vi "OpenTextFile.vi"(4 "Sequence Context":T1) -> (0 "error out":errorcluster, 1 "Test Data":T2 {"Numeric Measurement" format="%.2f"})   [LabVIEW 2012]
uses:
  <vilib>/addons/TestStand/_TSLegacy.llb/LabVIEW Test - Test Data.ctl
  <vilib>/addons/TestStand/_TSLegacy.llb/LabVIEW Test - Sequence Context.ctl
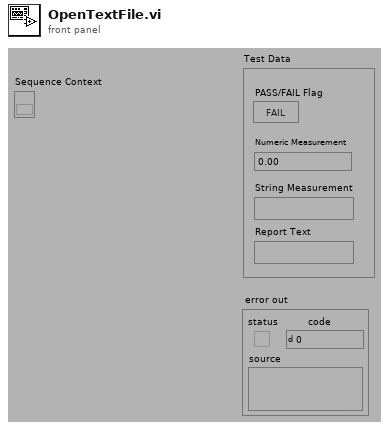
[diagram p1: front panel]
types:
  T1 = typedef "LabVIEW Test - Sequence Context.ctl" = refnum<k7>
  T2 = typedef "LabVIEW Test - Test Data.ctl" = cluster{"PASS/FAIL Flag":bool, "Numeric Measurement":dbl, "String Measurement":string, "Report Text":string}
  T3 = enum16{"open", "open or create", "create or replace", "create", "open (read only)"}
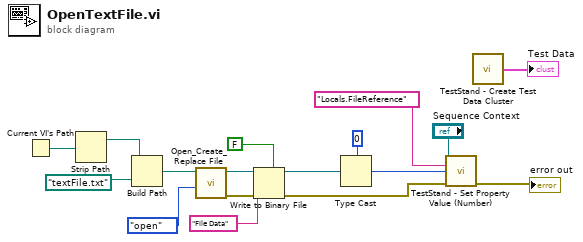
[diagram p0: block diagram]
diagram:
  n1 = Current VI's Path() -> (path=w9:path)
  n2 = Strip Path(path=w9) -> (stripped path=w7:path)  [unwired: 1 out]
  n3 = Build Path(base path=w7, name or relative path=path "textFile.txt" ("file path")) -> (appended path=w5:path)
  n4 = call <vilib>:"Open_Create_Replace File.vi"("function (open:0)"=T3."open", "file path"=w5) -> ("error out"=w3:errorcluster, "refnum"=w4:refnum<file>)  [unwired: 4 in, 4 out]
  n5 = Write to Binary File(file (use dialog)=w4, data="File Data", error in=w3, 5:FALSE ("prepend array or string size? (T)")) -> (refnum out=w12:refnum<file>, error out=w11:errorcluster)  [unwired: 3 out]
  n6 = Type Cast(type=u32 0, x=w12) -> (*(type *) &x=w15:u32)
  n7 = call <vilib>:"TestStand - Set Property Value (Number).vi"("Sequence Context In"="Sequence Context", "Lookup String"="Locals.FileReference", "New Value"=w15, "error in (no error)"=w11) -> ("error out"=→"error out":errorcluster)  [unwired: 1 in, 10 out]
  n8 = call <vilib>:"TestStand - Create Test Data Cluster.vi"() -> ("Test Data"=→"Test Data":T2)  [unwired: 4 in]
